vi "Use Case3.vi"() -> ()   [LabVIEW 2021, in "uCanDriver.lvlib" / "uCAN.lvclass"]
uses:
  uCAN.lvclass
  typedefs/frame.ctl
  typedefs/bitrates.ctl
panel:
  in  "Trace length":u64=100
  out "Table Control":string[][](table)
  in  "New Frame":T1
  in  "Bitrates":T2=enum."500 kbit/s"
  in  "COM port":refnum<visa-resource-name>="COM9"
  in  "Transmit Frame":bool
  in  "stop":bool
  out "Received Frames":T1[](array[typedef]) {"Data" format="%.0x"}
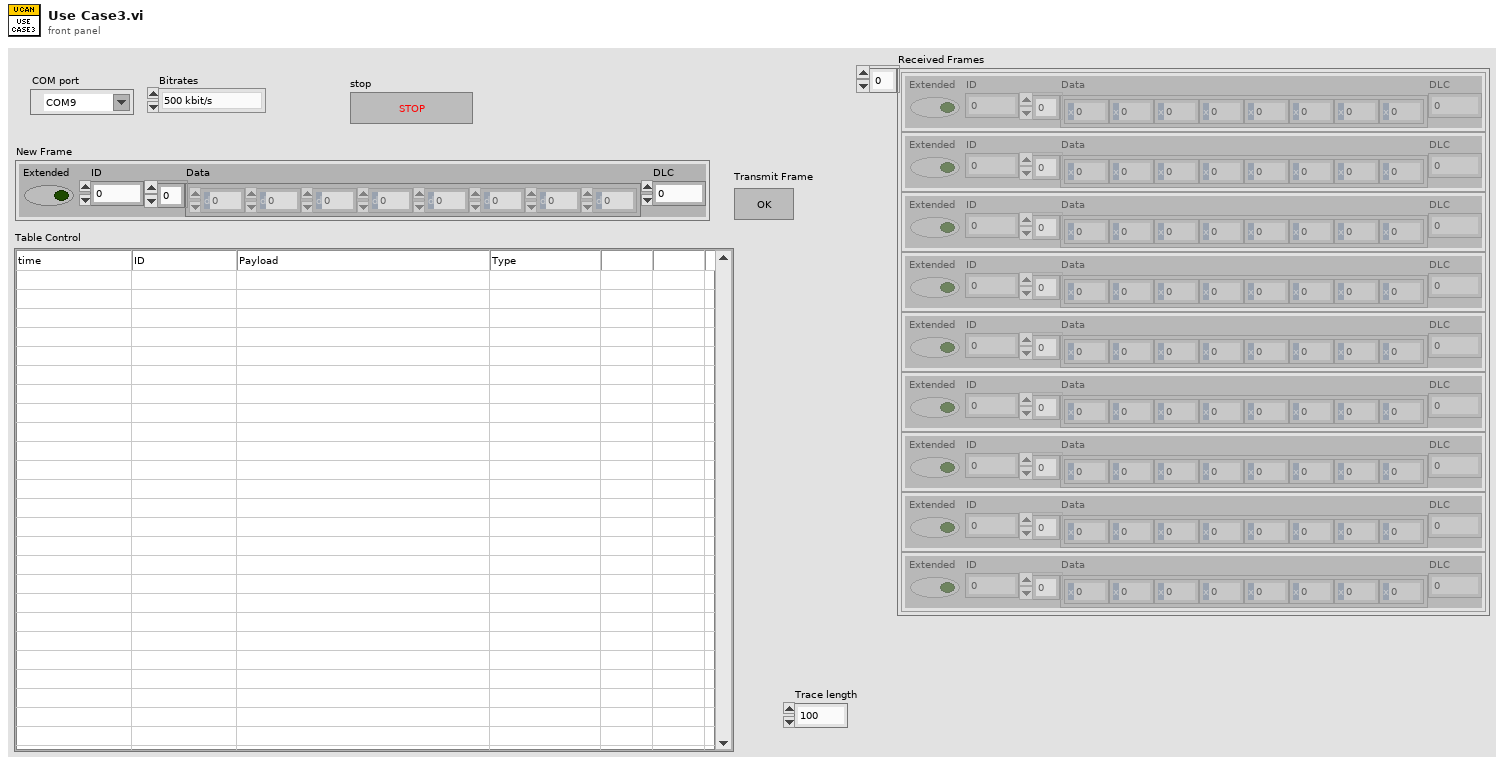
[diagram p1: front panel]
types:
  T1 = typedef "uCanDriver.lvlib/uCAN.lvclass/frame.ctl" = cluster{"Extended":bool, "ID":u32, "Data":u8[], "DLC":u8}
  T2 = typedef "uCanDriver.lvlib/uCAN.lvclass/bitrates.ctl" = enum16{"100 kbit/s", "125 kbit/s", "250 kbit/s", "500 kbit/s", "800 kbit/s", "1 Mbit/s"}
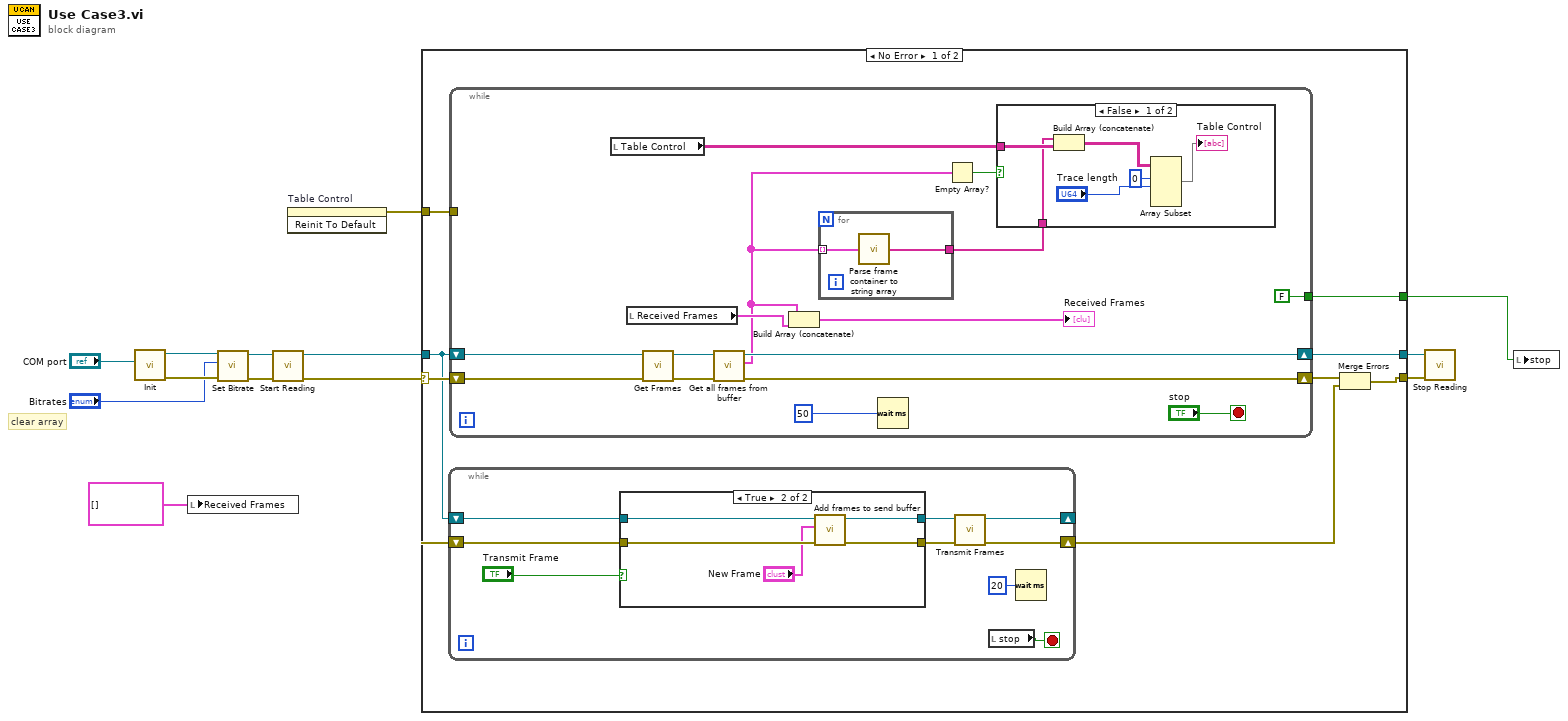
[diagram p0: block diagram]
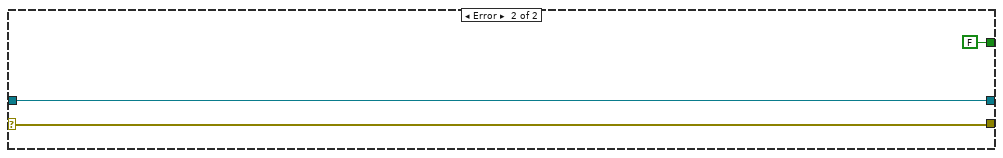
[diagram p4: hidden frame]
diagram:
  # "clear array"
  n1 = call "Init.vi"("COM port"="COM port") -> ("error out"=w11:errorcluster, "uCAN out"=w12:refnum<class "uCAN.lvclass">)  [unwired: 9 in]
  n2 = local write "Received Frames"(T1[] [] ("Received Frames Array")) -> ()
  n3 = call "Set Bitrate.vi"("error in (no error)"=w11, "Bitrates"="Bitrates", "uCAN in"=w12) -> ("error out"=w6:errorcluster, "uCAN out"=w4:refnum<class "uCAN.lvclass">)  [unwired: 7 in]
  n4 = call "Start Reading.vi"("error in (no error)"=w6, "uCAN in"=w4) -> ("error out"=w5:errorcluster, "uCAN out"=w3:refnum<class "uCAN.lvclass">)  [unwired: 8 in]
  n5 = invoke on="Table Control" class="Tbl (strict)" method="Reinit To Default"() -> (error out=w2:errorcluster)  [unwired: 3 in, 2 out]
  n6 = case shown="No Error" w5 {
    selector: w5 -> [w17 w63]
    tunnel: [w21 w62] -> w9
    tunnel: [w19 w63] -> w7
    tunnel: w3 -> [w16 w62]
    tunnel: w2 -> [w15 _]
    tunnel: [w14 FALSE ("stop")] -> w1
    frame No Error {
      n7 = while {
        shift-right: [w47] -> _
        shift-left: w16 -> [w53]
        shift-right: [w49] -> w18
        shift-left: w17 -> [w52]
        stop <- w46 stop-if-true
        n8 = case shown="True" "Transmit Frame" {
          tunnel: w53 -> [w55 w60]
          tunnel: w52 -> [w54 w59]
          tunnel: [w54 w58] -> w51
          tunnel: [w55 w57] -> w48
          frame False {
          }
          frame True {
            n9 = call "Add frames to send buffer.vi"("error in (no error)"=w59, "New Frame"="New Frame", "uCAN in"=w60) -> ("error out"=w58:errorcluster, "uCAN out"=w57:refnum<class "uCAN.lvclass">)  [unwired: 7 in]
          }
        }
        n10 = call "Transmit Frames.vi"("error in (no error)"=w51, "uCAN in"=w48) -> ("error out"=w49:errorcluster, "uCAN out"=w47:refnum<class "uCAN.lvclass">)  [unwired: 8 in]
        n11 = local read "stop"() -> (w46:bool)
        n12 = Wait (ms)(milliseconds to wait=u32 20) -> ()  [unwired: 1 out]
      }
      n13 = while {
        shift-right: [w32] -> w21
        shift-left: w16 -> [w36]
        shift-right: [w31] -> w20
        shift-left: w17 -> [w35]
        tunnel: w15 -> [_]
        tunnel: [FALSE ("stop")] -> w14
        stop <- "stop" stop-if-true
        n14 = local read "Table Control"() -> (w26:string[][])
        n15 = local read "Received Frames"() -> (w27:T1[])
        n16 = call "Get Frames.vi"("error in (no error)"=w35, "uCAN in"=w36) -> ("error out"=w34:errorcluster, "uCAN out"=w33:refnum<class "uCAN.lvclass">)  [unwired: 7 in, 1 out]
        n17 = call "Get all frames from buffer.vi"("error in (no error)"=w34, "uCAN in"=w33) -> ("error out"=w31:errorcluster, "Received Frames Array"=w22:T1[], "uCAN out"=w32:refnum<class "uCAN.lvclass">)  [unwired: 7 in]
        n18 = Build Array (concatenate)(w22, w27) -> (→"Received Frames":T1[])
        n19 = for {
          tunnel: [w38] -> w23
          tunnel: w22 -> [w37] mode=indexing
          n20 = call "Parse frame container to string array.vi"("Frame"=w37) -> ("String array"=w38:string[])
        }
        n21 = Wait (ms)(milliseconds to wait=u32 50) -> ()  [unwired: 1 out]
        n22 = Empty Array?(array=w22) -> (empty?=w25:bool)
        n23 = case shown="False" w25 {
          tunnel: w26 -> [w44 _]
          tunnel: w23 -> [w43 _]
          frame False {
            n24 = Build Array (concatenate)(w43, w44) -> (w40:string[][])
            n25 = Array Subset(array=w40, index (row)=0 ("index"), length (row)="Trace length") -> (→"Table Control":string[][])  [unwired: 2 in]
          }
          frame True {
          }
        }
      }
      n26 = Merge Errors(w20, w18) -> (w19:errorcluster)
    }
    frame Error {
    }
  }
  n27 = call "Stop Reading.vi"("error in (no error)"=w7, "uCAN in"=w9) -> ()  [unwired: 8 in, 2 out]
  n28 = local write "stop"(w1) -> ()
